vi "anCLASS.vi"(7 "Set? (f)":bool, 11 "SpecAnPlugins.lvlib In":refnum<class "SpecAnBase.lvclass">) -> (3 "SpecAnPlugins.lvlib Out":refnum<class "SpecAnBase.lvclass">)   [LabVIEW 2018, in "SpecAnModule.lvlib"]
uses:
  SpecAnModule.lvlib
  SpecAnPlugins/SpecAnBaseClass/SpecAnBase.lvclass
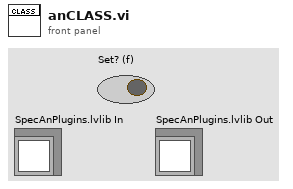
[diagram p1: front panel]
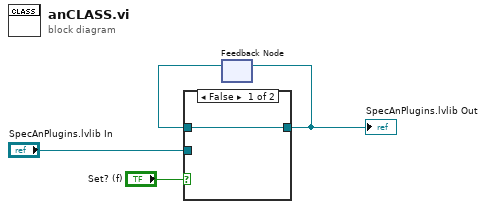
[diagram p0: block diagram]
diagram:
  n1 = feedback #1() -> (w3:refnum<class "SpecAnBase.lvclass">)  [unwired: 1 in]
  n2 = case shown="False" "Set? (f)" {
    tunnel: "SpecAnPlugins.lvlib In" -> [_ w6]
    tunnel: [w5 w6] -> w1
    tunnel: w3 -> [w5 _]
    frame False {
    }
    frame True {
    }
  }
  "SpecAnPlugins.lvlib Out" <- w1
  n3 = feedback-in #1(w1) -> ()
